vi "#kaputt-#marchePas-#Scheisscaca-#wtfBordel-MonitoringSemiOp.vi"() -> ()   [LabVIEW 2013]
panel:
  in  "Envoi":bool
  in  "data in":string
  out "?":bool
  in  "Afficher caractères reçus":bool
  in  "Log":bool
  out "error out":errorcluster
  out "Caractères reçus":string
  in  "Mode":T1(ring)=enum."CRLF"
  in  "?":bool
  in  "Tab Control":T2(tab)
  out "Signal Camera     ->    Fronts détectés":dbl[](graph)
  out "Signal Camera    ->  original":dbl[](graph)
  out "Moyenne":dbl
  out "?":dbl
  out "Position Servo":dbl(knob) scale=0.0..10.0
  out "Effective droite":dbl
  out "Consigne droite":dbl
  out "Effective gauche":dbl
  out "Consigne gauche":dbl
  out "Vitesse roue arrière droite [m/s]":dbl(knob) scale=0.0..10.0
  out "Vitesse roue arrière gauche [m/s]":dbl(knob) scale=0.0..10.0
  in  "PID 3.3":dbl
  in  "PID 3.2":dbl
  in  "PID Direction":dbl
  in  "ABS":bool
  out "?":bool
  in  "PID vitesse":bool
  out "?":bool
  out "?":bool
  out "Array":bool[](array[boolean])
  in  "PID 2.3":i8
  in  "PID 2.2":i8
  in  "PID Léger":i8
  in  "PID 1.3":i8
  in  "PID 1.2":i8
  in  "PID Fort":i8
  # "Fort"
  # "Léger"
  # "Droite"
  # "Gauche"
  # "Fin"
  # "Perte Ligne"
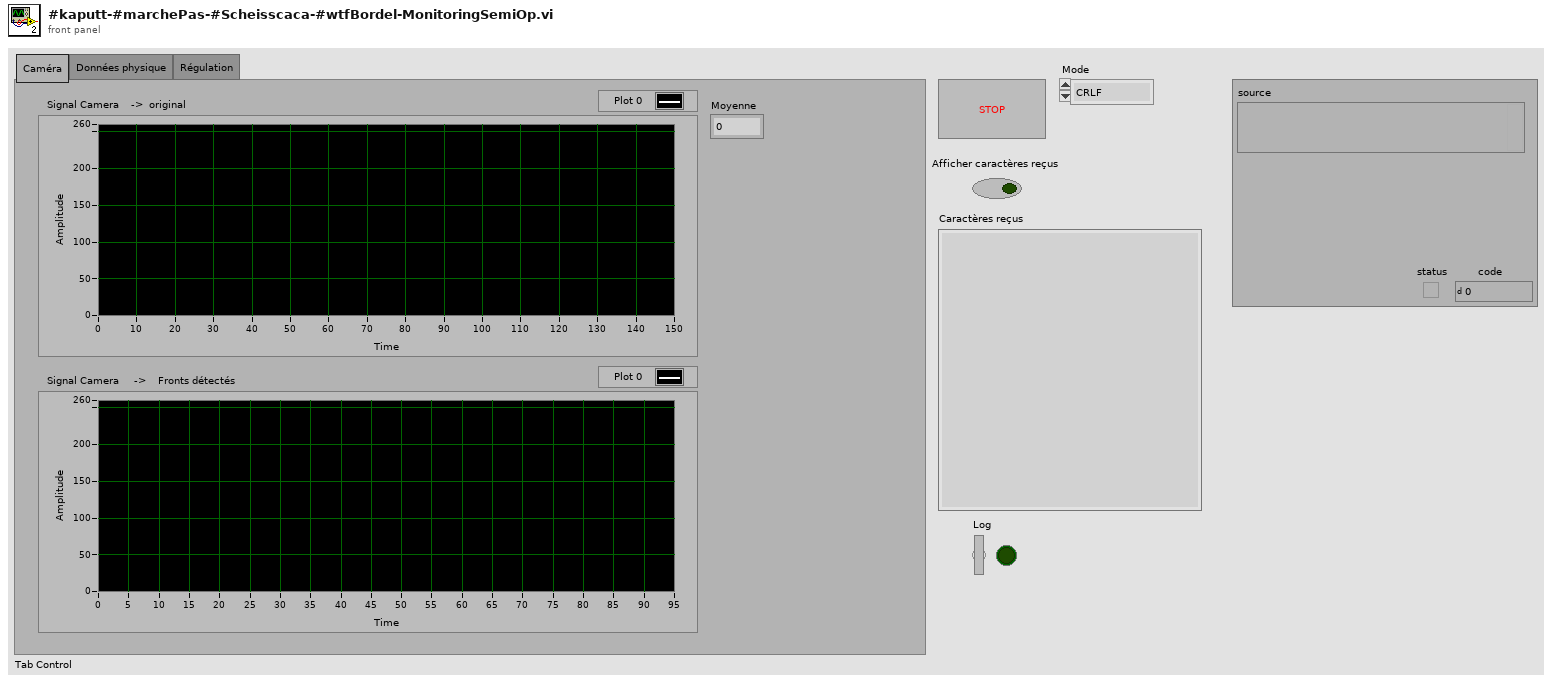
[diagram p1: front panel]
types:
  T1 = enum16{"Standard", "Buffered", "CRLF", "Immediate"}
  T2 = enum32{"Caméra", "Données physique", "Régulation"}
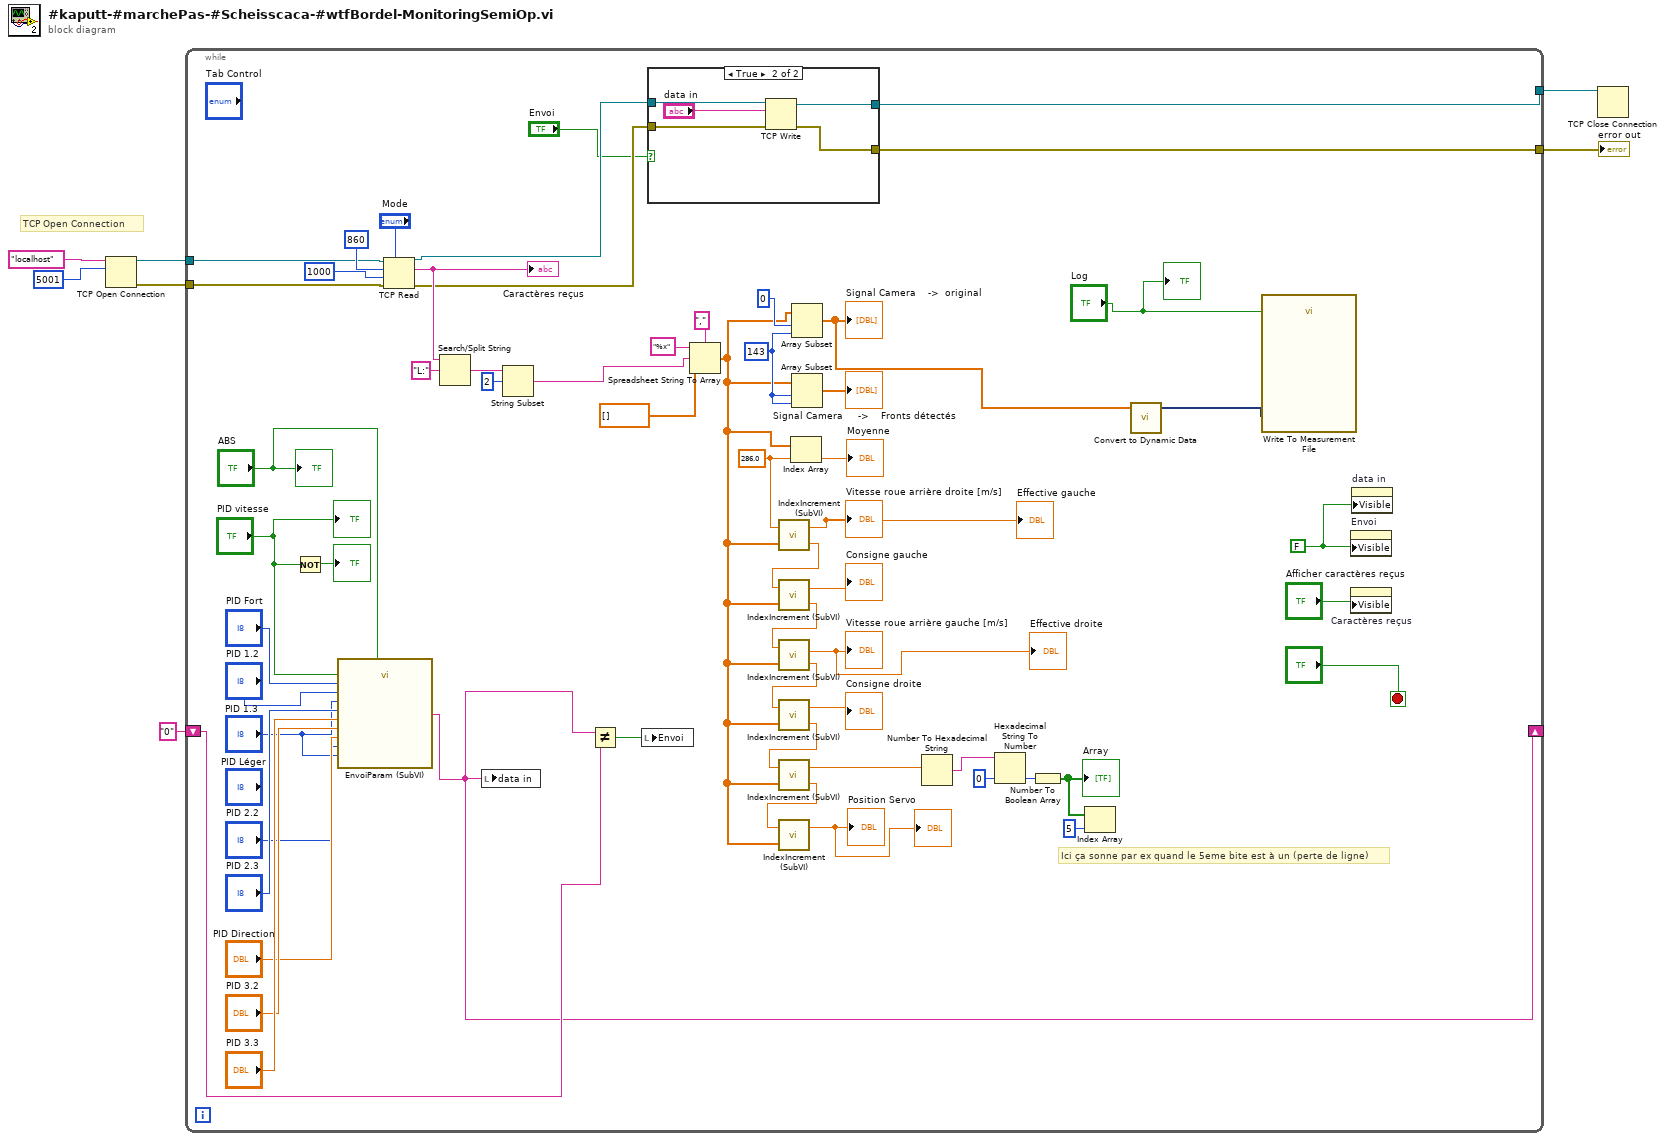
[diagram p0: block diagram]
diagram:
  # "TCP Open Connection"
  n1 = TCP Open Connection(address="localhost", remote port or service name=u16 5001) -> (connection ID=w5:refnum<k5>, error out=w4:errorcluster)  [unwired: 3 in]
  n2 = while {
    tunnel: w5 -> [w41]
    tunnel: w4 -> [w54]
    tunnel: [w39] -> w3
    tunnel: [w37] -> w2
    shift-right: [w10] -> _
    shift-left: "0" -> [w34]
    stop <- "?" stop-if-true
    w35 = FALSE
    w32 = 286.0 ("x")
    w53 = 143 ("length")
    # "Ici ça sonne par ex quand le 5eme bite est à un (perte de ligne)"
    n3 = Not(x="PID vitesse") -> (.not. x?=→"?":bool)
    n4 = call "EnvoiParam (SubVI).vi"("PID 3.3"="PID 3.3", "PID 3.2"="PID 3.2", "PID Direction"="PID Direction", "PID 2.3"="PID 2.3", "PID 2.2"="PID 2.2", "PID Léger"="PID 1.3", "PID 1.3"="PID 1.3", "PID 1.2"="PID 1.2", "PID Fort"="PID Fort", "PID vitesse"="PID vitesse", "ABS"="ABS") -> ("String"=w10:string)
    n5 = TCP Read(connection ID=w41, bytes to read=860, error in (no error)=w54, 7:"Mode", 9:1000 ("timeout ms (25000)")) -> (connection ID out=w40:refnum<k5>, data out=w62:string, error out=w38:errorcluster)
    "Caractères reçus" <- w62
    n6 = Search/Split String(string=w62, search string/char (-)="L:") -> (match + rest of string=w60:string)  [unwired: 1 in, 2 out]
    n7 = local write "data in"(w10) -> ()
    n8 = String Subset(string=w60, offset (0)=2) -> (substring=w61:string)  [unwired: 1 in]
    n9 = Not Equal?(x=w10, y=w34) -> (x != y?=w33:bool)
    n10 = local write "Envoi"(w33) -> ()
    n11 = case shown="True" "Envoi" {
      tunnel: w40 -> [w69 w74]
      tunnel: [w69 w73] -> w39
      tunnel: w38 -> [w68 w72]
      tunnel: [w68 w71] -> w37
      frame False {
      }
      frame True {
        n12 = TCP Write(connection ID=w74, data in="data in", error in (no error)=w72) -> (connection ID out=w73:refnum<k5>, error out=w71:errorcluster)  [unwired: 1 in, 1 out]
      }
    }
    n13 = Spreadsheet String To Array(delimiter (Tab)=",", format string="%x", spreadsheet string=w61, array type (2D Dbl)=dbl[] []) -> (array=w21:dbl[])
    n14 = call "IndexIncrement (SubVI).vi"("array type (2D Dbl)"=w21, "Index"=w32) -> ("Index+1"=w30:dbl, "Out"=→"Vitesse roue arrière droite [m/s]" →"Effective gauche":dbl)
    n15 = call "IndexIncrement (SubVI).vi"("array type (2D Dbl)"=w21, "Index"=w30) -> ("Index+1"=w29:dbl, "Out"=→"Consigne gauche":dbl)
    n16 = call "IndexIncrement (SubVI).vi"("array type (2D Dbl)"=w21, "Index"=w29) -> ("Index+1"=w28:dbl, "Out"=→"Vitesse roue arrière gauche [m/s]" →"Effective droite":dbl)
    n17 = call "IndexIncrement (SubVI).vi"("array type (2D Dbl)"=w21, "Index"=w28) -> ("Index+1"=w27:dbl, "Out"=→"Consigne droite":dbl)
    n18 = call "IndexIncrement (SubVI).vi"("array type (2D Dbl)"=w21, "Index"=w27) -> ("Index+1"=w26:dbl, "Out"=w23:dbl)
    n19 = call "IndexIncrement (SubVI).vi"("array type (2D Dbl)"=w21, "Index"=w26) -> ("Out"=→"Position Servo" →"?":dbl)  [unwired: 1 out]
    n20 = Index Array(array=w21, index=w32) -> (element=→"Moyenne":dbl)
    n21 = Array Subset(array=w21, index=0, length=w53) -> (w46:dbl[])
    "Signal Camera    ->  original" <- w46
    n22 = Array Subset(array=w21, index=w53, length=w53) -> (→"Signal Camera     ->    Fronts détectés":dbl[])
    n23 = Number To Hexadecimal String(2:w23) -> (0:w49:string)  [unwired: 1 in]
    n24 = Hexadecimal String To Number(string=w49, default (0uL)=u8 0 ("default (0 U32)")) -> (number=w50:u8)  [unwired: 1 in, 1 out]
    n25 = Number To Boolean Array(number=w50) -> (Boolean array=w48:bool[])
    "Array" <- w48
    n26 = Index Array(array=w48, index=5) -> ()  [unwired: 1 out]
    n27 = call "Convert to Dynamic Data"("Array"=w46) -> ("Dynamic Data Type"=w44:dynamicdata)  [unwired: 3 in]
    n28 = call "Write To Measurement File"("Signals"=w44, "Enable"="Log") -> ()  [unwired: 15 in, 3 out]
    n29 = property on="Envoi" class="Bool (strict)"("Visible"=w35) -> ()  [unwired: 2 in, 2 out]
    n30 = property on="Caractères reçus" class="Str"("Visible"="Afficher caractères reçus") -> ()  [unwired: 2 in, 2 out]
    n31 = property on="data in" class="Str"("Visible"=w35) -> ()  [unwired: 2 in, 2 out]
    "?" <- "ABS"
    "?" <- "PID vitesse"
    "?" <- "Log"
  }
  "error out" <- w2
  n32 = TCP Close Connection(connection ID=w3) -> ()  [unwired: 2 in, 2 out]
